vi "Update UI Values.vi"(8 "error in (no error)":errorcluster, 9 "This VI":refnum<vi>, 10 "Controls Value":variant, 11 "PanelManager in":refnum<class "PanelManager.lvclass">) -> (0 "error out":errorcluster, 3 "PanelManager out":refnum<class "PanelManager.lvclass">)   [LabVIEW 2015, in "PanelManager.lvclass"]
uses:
  PanelManager.lvclass
  <vilib>/Utility/traverseref.llb/TRef TravTarget.ctl
  <vilib>/Utility/traverseref.llb/VI Scripting - Traverse.lvlib
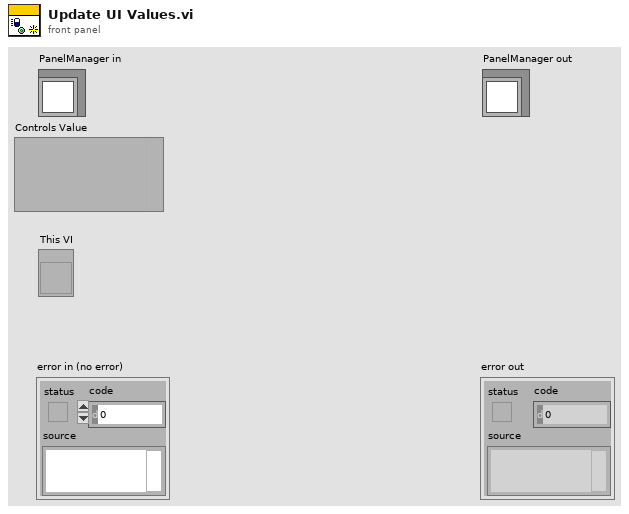
[diagram p1: front panel]
types:
  T1 = typedef "TRef TravTarget.ctl" = enum16{"FP", "BD", "Other"}
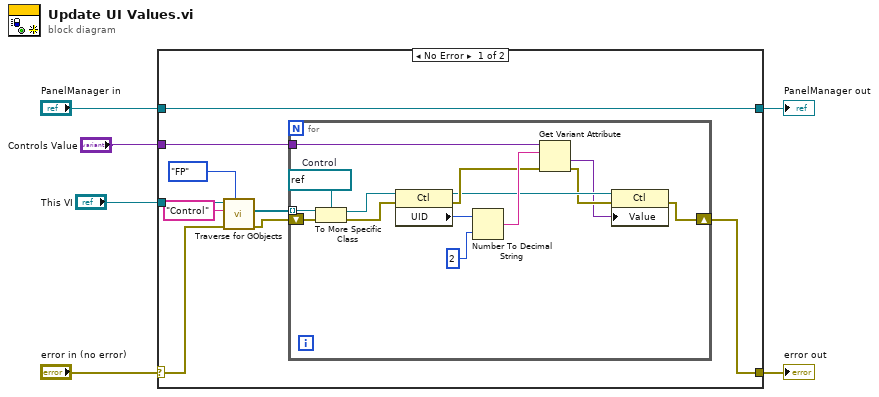
[diagram p0: block diagram]
diagram:
  n1 = case shown="No Error" "error in (no error)" {
    selector: "error in (no error)" -> [w13 w31]
    tunnel: [w8 w31] -> w5
    tunnel: [w9 w30] -> w3
    tunnel: "PanelManager in" -> [w9 w30]
    tunnel: "This VI" -> [w15 _]
    tunnel: "Controls Value" -> [w7 _]
    frame No Error {
      n2 = call <vilib>:"Traverse for GObjects.vi"("Traverse Target"=TRef_TravTarget."FP", "error in (no error)"=w13, "Class Name"="Control", "VI Refnum"=w15) -> ("error out"=w10:errorcluster, "References"=w11:refnum<vi>[])  [unwired: 4 in, 2 out]
      n3 = for {
        tunnel: w11 -> [w29] mode=indexing
        tunnel: w7 -> [w24]
        shift-right: [w16] -> w8
        shift-left: w10 -> [w28]
        w27 = refnum<vi> refnum  # Control
        n4 = To More Specific Class(target class=w27, reference=w29, error in=w28) -> (specific class reference=w26:refnum<vi>, error out=w25:errorcluster)
        n5 = property class="Ctl"(reference=w26, error in=w25) -> (reference out=w19:refnum<vi>, error out=w20:errorcluster, "UID"=w23:i32)
        n6 = Number To Decimal String(number=w23, width (-)=i16 2) -> (decimal integer string=w21:string)
        n7 = Get Variant Attribute(Variant=w24, name=w21, error in=w20) -> (value=w17:variant, error out=w18:errorcluster)  [unwired: 1 in, 2 out]
        n8 = property class="Ctl"(reference=w19, error in=w18, "Value"=w17) -> (error out=w16:errorcluster)  [unwired: 1 out]
      }
    }
    frame Error {
    }
  }
  "error out" <- w5
  "PanelManager out" <- w3
